vi "create tag channels.vi"(6 "channel classification (input data)":T1, 9 "data type":T2, 10 "tag name":string) -> (3 "channel":refnum<class "TBM channel.lvclass">)   [LabVIEW 2013, in "current tag file io module configuration.lvclass"]
uses:
  current tag file io module configuration.lvclass
  <vilib>/NI/Tag Bus/tag/Data Type.ctl
  <vilib>/NI/Tag Bus Module Framework/channel/TBM channel.lvclass
  <vilib>/NI/Tag Bus Module Framework/channel/channel classification.ctl
  <vilib>/NI/Tag Bus/tag/tag descriptor.lvclass
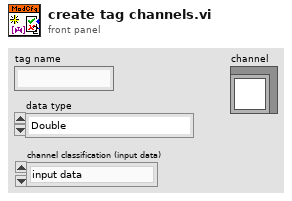
[diagram p1: front panel]
types:
  T1 = typedef "TBM channel.lvclass/channel classification.ctl" = enum16{"input data", "output data", "processing parameter", "processing result"}
  T2 = typedef "tag bus.lvlib/tag descriptor.lvclass/Data Type.ctl" = enum16{"Double", "Single", "I64", "I32", "I16", "I8", "U64", "U32", "U16", "U8", "Boolean", "String", "Array of Double", "Array of Single", "Array of I64", "Array of I32", "Array of I16", "Array of I8", "Array of U64", "Array of U32", "Array of U16", "Array of U8", "Array of Boolean", "Array of String"}
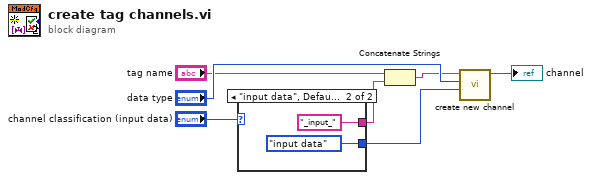
[diagram p0: block diagram]
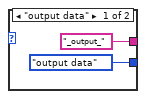
[diagram p2: hidden frame]
diagram:
  n1 = case shown="\"input data\", Default" "channel classification (input data)" {
    tunnel: ["_output_" ("string") "_input_" ("string")] -> w1
    tunnel: [channel_classification."output data" ("channel classification") channel_classification."input data" ("channel classification")] -> w2
    frame "output data" {
    }
    frame "input data", Default {
    }
  }
  n2 = Concatenate Strings("tag name", w1) -> (w4:string)
  n3 = call <vilib>:"create new channel.vi"("channel classification"=w2, "data type"="data type", "channel name"=w4) -> ("channel"=→"channel":refnum<class "TBM channel.lvclass">)  [unwired: 8 in]
